vi "is_finished.vi"(8 "error in (no error)":errorcluster, 11 "ImagingModeMG090624Camera in":refnum<class "ImagingModeMG090624Camera.lvclass">) -> (0 "error out":errorcluster, 2 "finished?":bool[](array[boolean]), 3 "ImagingModeMG090624Camera out":refnum<class "ImagingModeMG090624Camera.lvclass">)   [LabVIEW 2010, in "ImagingModeMG090624Camera.lvclass"]
uses:
  ImagingModeMG090624Camera.lvclass
  ImagingModeMG090624Camera.lvclass/ImagingModeMG090624Camera.ctl
panel:
  # "element 0: is sweep finished?\n(further elements might be defined by overriding methods)"
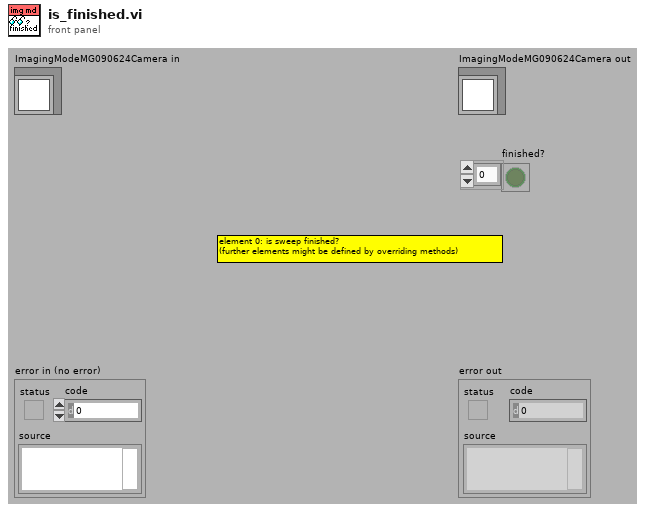
[diagram p1: front panel]
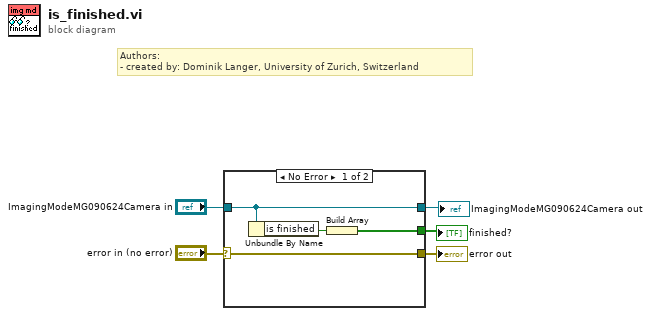
[diagram p0: block diagram]
diagram:
  # "Authors: \n- created by: Dominik Langer, University of Zurich, Switzerland"
  n1 = case shown="No Error" "error in (no error)" {
    selector: "error in (no error)" -> [w9 w10]
    tunnel: "ImagingModeMG090624Camera in" -> [w6 w11]
    tunnel: [w9 w10] -> w3
    tunnel: [w7 _] -> w2
    tunnel: [w6 w11] -> w1
    frame No Error {
      n2 = Unbundle By Name(w6) -> ("is finished"=w8:bool)
      n3 = Build Array(w8) -> (w7:bool[])
    }
    frame Error {
    }
  }
  "error out" <- w3
  "ImagingModeMG090624Camera out" <- w1
  "finished?" <- w2
